vi "detect_dropped_frames.vi"(11 "Frame Number":i64) -> (2 "% dropped frames":dbl, 3 "Dropped frames (per frame)":dbl)   [LabVIEW 2010]
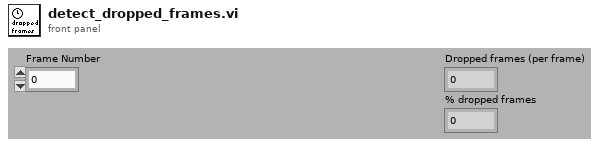
[diagram p1: front panel]
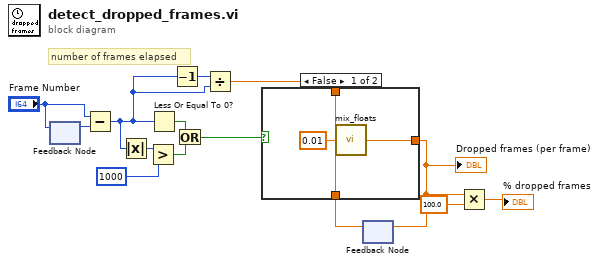
[diagram p0: block diagram]
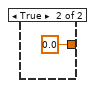
[diagram p2: hidden frame]
diagram:
  # "number of frames elapsed"
  n1 = feedback-in #1("Frame Number") -> ()
  n2 = feedback #1() -> (w14:i64)  [unwired: 1 in]
  n3 = Subtract(x="Frame Number", y=w14) -> (x-y=w2:i64)
  n4 = Absolute Value(x=w2) -> (abs(x)=w12:i64)
  n5 = Greater?(x=w12, y=i64 1000) -> (0:w10:bool)
  n6 = Less Or Equal To 0?(x=w2) -> (x <= 0?=w9:bool)
  n7 = Decrement(x=w2) -> (x-1=w3:i64)
  n8 = Or(x=w9, y=w10) -> (x .or. y?=w8:bool)
  n9 = Divide(x=w3, y=w2) -> (x/y=w1:dbl)
  n10 = feedback #2() -> (w7:dbl)  [unwired: 1 in]
  n11 = case shown="False" w8 {
    tunnel: w1 -> [w17 _]
    tunnel: [w16 0.0 ("alpha * x + (1-alpha) * y")] -> w6
    tunnel: w7 -> [w15 _]
    frame False {
      n12 = call "mix_floats.vi"("y"=w15, "alpha"=0.01, "x"=w17) -> ("alpha * x + (1-alpha) * y"=w16:dbl)
    }
    frame True {
    }
  }
  "Dropped frames (per frame)" <- w6
  n13 = feedback-in #2(w6) -> ()
  n14 = Multiply(x=w6, y=100.0) -> (x*y=→"% dropped frames":dbl)
